vi "Push_Data_via_Public_Client.vi"(5 "Archive File?":bool[](array[boolean]), 6 "application reference":refnum<vi>, 7 "error in (no error)":errorcluster, 8 "Running on Server?":bool, 10 "Path of Files relative to EnFlo Data Root":path[](array[path])) -> (0 "error out":errorcluster, 3 "Error String":string)   [LabVIEW 2016]
uses:
  Anemometry/Anemometry Sub Vis/Globals/Constants_global.vi
  Sub VIs/Harvest_Global.vi
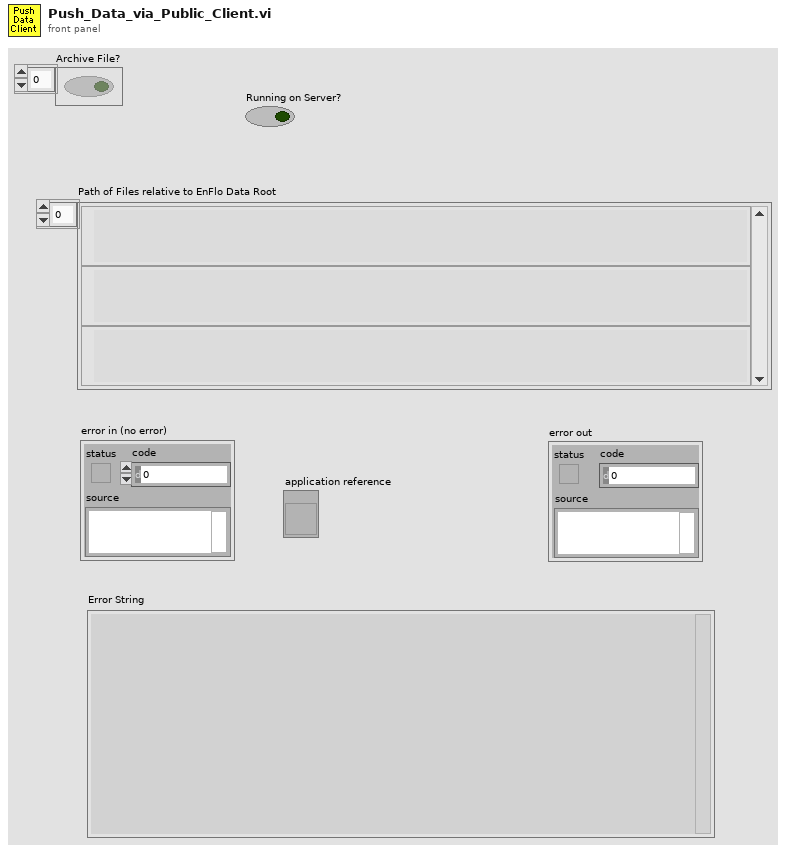
[diagram p1: front panel]
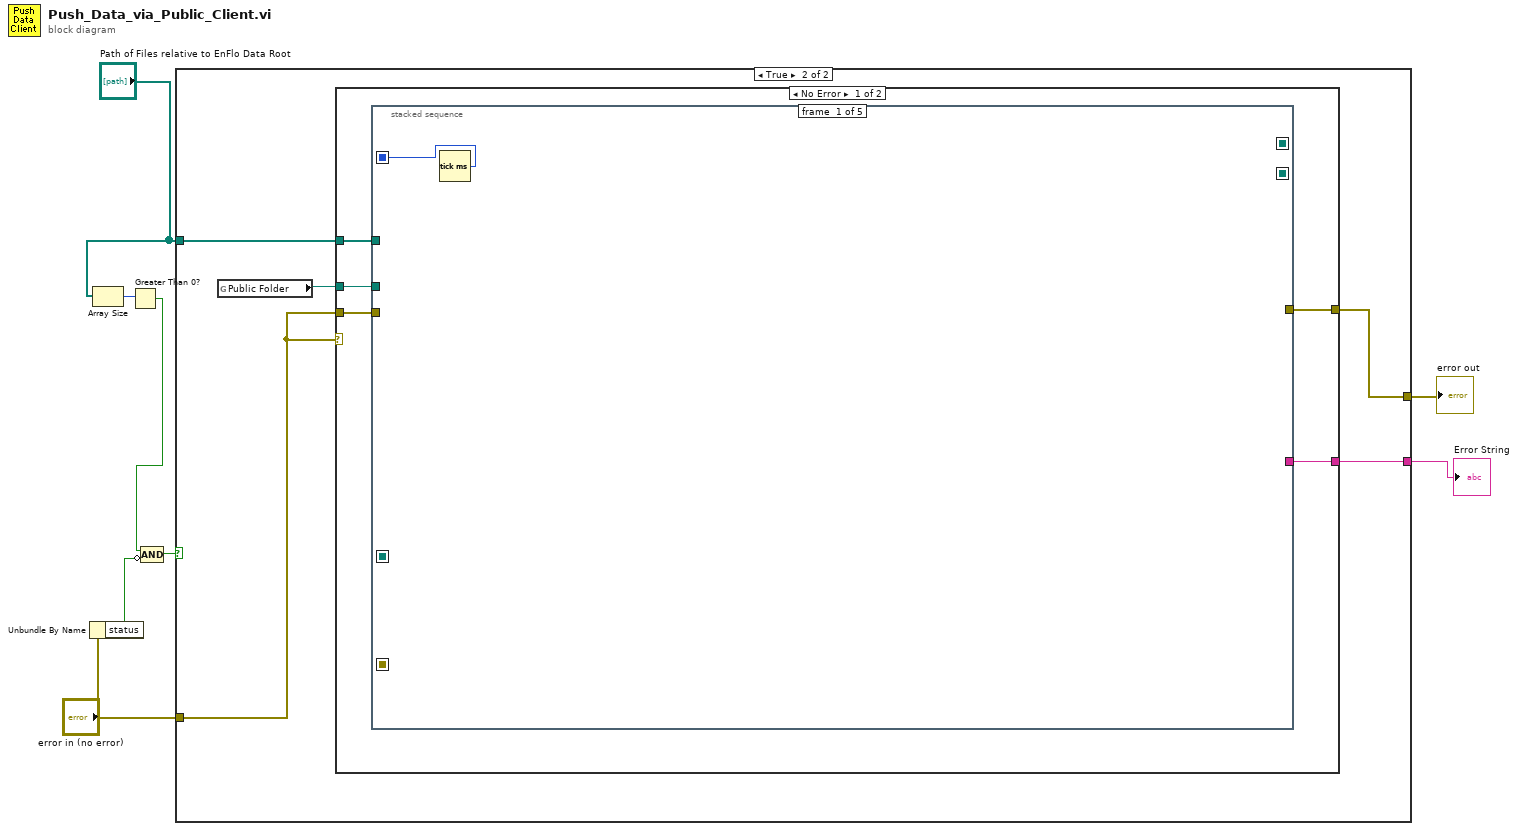
[diagram p0: block diagram]
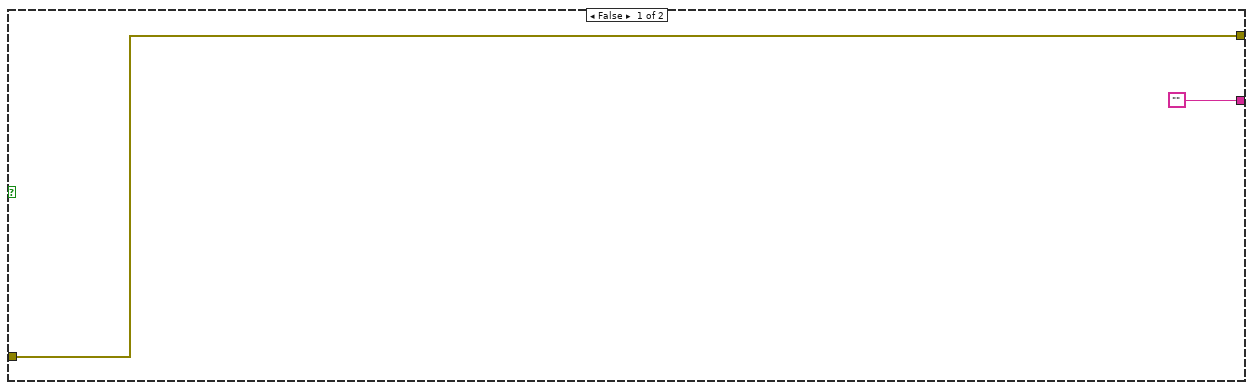
[diagram p2: hidden frame]
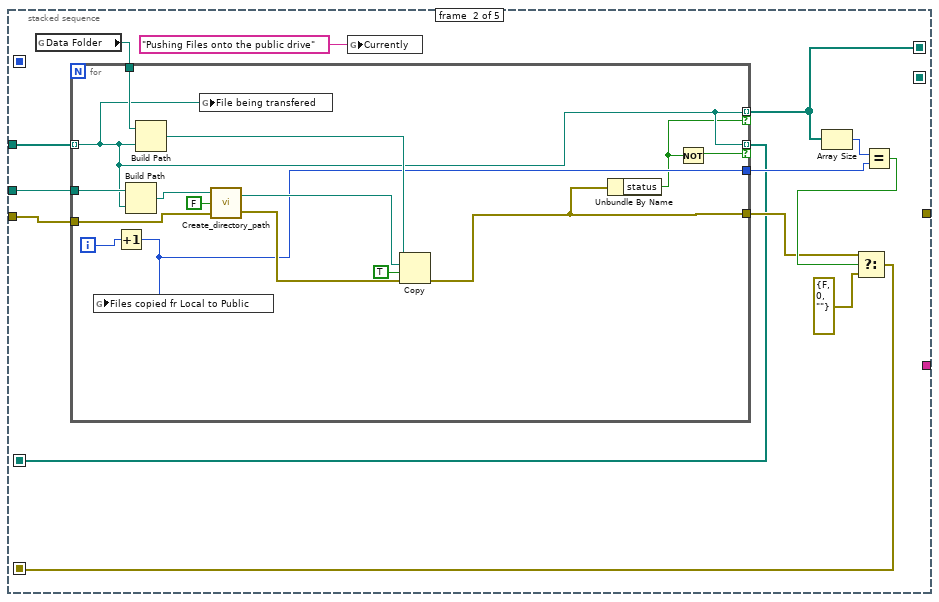
[diagram p3: hidden frame]
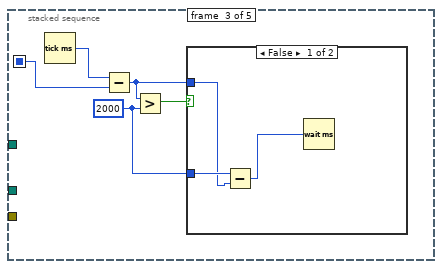
[diagram p4: hidden frame]
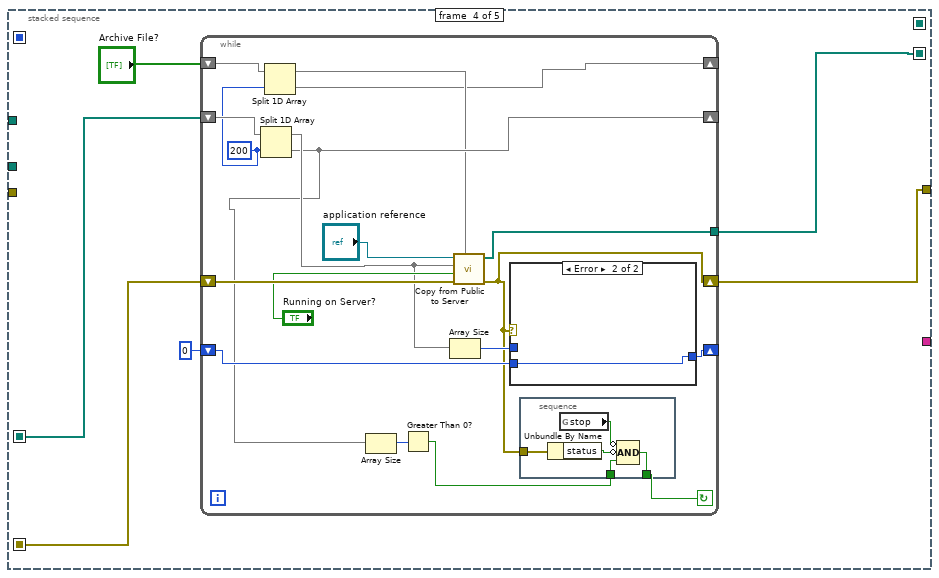
[diagram p6: hidden frame]
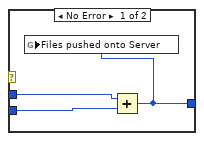
[diagram p7: hidden frame]
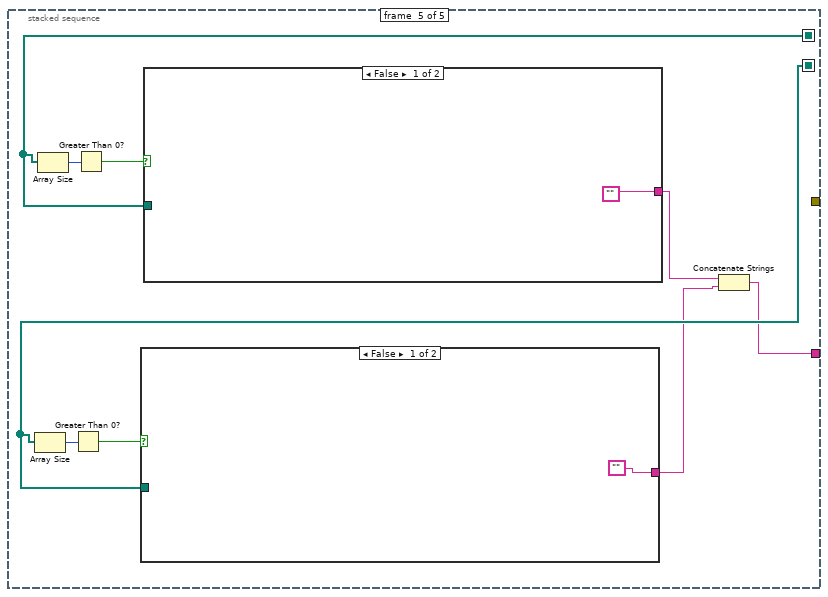
[diagram p8: hidden frame]
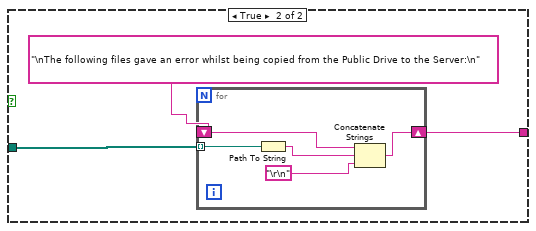
[diagram p9: hidden frame]
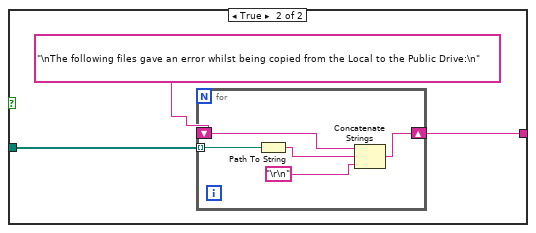
[diagram p10: hidden frame]
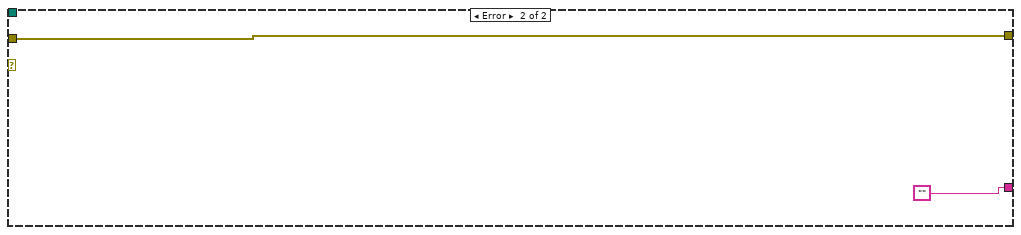
[diagram p11: hidden frame]
diagram:
  n1 = Unbundle By Name("error in (no error)") -> ("status"=w3:bool)
  n2 = Array Size(array="Path of Files relative to EnFlo Data Root") -> (size(s)=w6:i32)
  n3 = Greater Than 0?(x=w6) -> (x > 0?=w4:bool)
  n4 = Compound Arithmetic op=AND(w4, invert w3) -> (w2:bool)
  n5 = case shown="True" w2 {
    tunnel: [w10 w12] -> w8
    tunnel: "error in (no error)" -> [w10 w15]
    tunnel: "Path of Files relative to EnFlo Data Root" -> [_ w13]
    tunnel: ["" w11] -> w1
    frame False {
    }
    frame True {
      n6 = global read "Constants_global.vi" "Public Folder"() -> (w14:path)
      n7 = case shown="No Error" w15 {
        tunnel: [w17 w119] -> w12
        tunnel: w15 -> [w18 w119]
        tunnel: w13 -> [w20 _]
        tunnel: w14 -> [w19 _]
        tunnel: [w16 ""] -> w11
        frame No Error {
          n8 = stacked-sequence {
            seq-local: [w21 _ _ _ _] -> [_ _ w53 _ _]
            seq-local: [_ w24 _ _ _] -> [_ _ _ w63 _]
            seq-local: [_ w23 _ _ _] -> [_ _ _ _ w99]
            seq-local: [_ w22 _ _ _] -> [_ _ _ w59 _]
            seq-local: [_ _ _ w58 _] -> [_ _ _ _ w94]
            tunnel: w20 -> [_ w33 _ _ _]
            tunnel: w19 -> [_ w32 _ _ _]
            tunnel: w18 -> [_ w31 _ _ _]
            tunnel: [_ _ _ w62 _] -> w17
            tunnel: [_ _ _ _ w91] -> w16
            frame #0 {
              n9 = Tick Count (ms)() -> (millisecond timer value=w21:u32)
            }
            frame #1 {
              n10 = global read "Constants_global.vi" "Data Folder"() -> (w34:path)
              n11 = for {
                tunnel: w34 -> [w43]
                tunnel: w33 -> [w37] mode=indexing
                tunnel: w32 -> [w47]
                tunnel: w31 -> [w44]
                tunnel: [w40] -> w25
                tunnel: [w37] -> w23 mode=indexing if=w36
                tunnel: [w39] -> w28
                tunnel: [w37] -> w22 mode=indexing if=w35
                i -> [w42]
                n12 = Increment(x=w42) -> (x+1=w39:i32)
                n13 = global write "Harvest_Global.vi" "Files copied fr Local to Public"(w39) -> ()
                n14 = Build Path(base path=w47, name or relative path=w37) -> (appended path=w48:path)
                n15 = Build Path(base path=w43, name or relative path=w37) -> (appended path=w49:path)
                n16 = global write "Harvest_Global.vi" "File being transfered"(w37) -> ()
                n17 = call "Create_directory_path.vi"("error in (no error)"=w44, "Dialog Box"=FALSE, "Path name"=w48) -> ("error out"=w45:errorcluster, "Path name Out"=w46:path)
                n18 = Copy(8:w45, 9:TRUE ("overwrite (F)"), 10:w46, 11:w49) -> (0:w40:errorcluster)  [unwired: 1 in, 2 out]
                n19 = Unbundle By Name(w40) -> ("status"=w36:bool)
                n20 = Not(x=w36) -> (.not. x?=w35:bool)
              }
              n21 = global write "Harvest_Global.vi" "Currently"("Pushing Files onto the public drive" ("Currently Running")) -> ()
              n22 = Array Size(array=w23) -> (size(s)=w29:i32)
              n23 = Equal?(x=w29, y=w28) -> (x = y?=w26:bool)
              n24 = Select(t=w25, s=w26, f=errorcluster {"status"=FALSE, "code"=0, "source"=""} ("error out")) -> (s? t:f=w24:errorcluster)
            }
            frame #2 {
              w51 = u32 2000 ("y")
              n25 = Tick Count (ms)() -> (millisecond timer value=w54:u32)
              n26 = Subtract(x=w54, y=w53) -> (x-y=w50:u32)
              n27 = Greater?(x=w50, y=w51) -> (0:w52:bool)
              n28 = case shown="False" w52 {
                tunnel: w51 -> [w57 _]
                tunnel: w50 -> [w56 _]
                frame False {
                  n29 = Subtract(x=w57, y=w56) -> (x-y=w55:u32)
                  n30 = Wait (ms)(milliseconds to wait=w55) -> ()  [unwired: 1 out]
                }
                frame True {
                }
              }
            }
            frame #3 {
              n31 = while {
                shift-right: [w73] -> w62
                shift-left: w63 -> [w81]
                shift-right: [w72] -> _
                shift-left: w59 -> [w78]
                shift-right: [w75] -> _
                shift-left: 0 -> [w74]
                shift-right: [w65] -> _
                shift-left: "Archive File?" -> [w68]
                tunnel: [w64] -> w58
                stop <- w69 continue-if-true
                w67 = 200 ("index")
                n32 = Split 1D Array(array=w78, index=w67) -> (first subarray=w77:path[], second subarray=w72:path[])
                n33 = Split 1D Array(array=w68, index=w67) -> (first subarray=w66:bool[], second subarray=w65:bool[])
                n34 = Array Size(array=w72) -> (size(s)=w71:i32)
                n35 = Greater Than 0?(x=w71) -> (x > 0?=w70:bool)
                n36 = Array Size(array=w77) -> (size(s)=w76:i32)
                n37 = call "Copy from Public to Server.vi"("Archive File?"=w66, "error in (no error)"=w81, "Running on Server?"="Running on Server?", "Path of Files relative to EnFlo Data Root"=w77, "Application in"="application reference") -> ("error out"=w73:errorcluster, "Problem Files"=w64:path[])  [unwired: 5 in]
                n38 = case shown="Error" w73 {
                  tunnel: w76 -> [w89 _]
                  tunnel: [w87 w90] -> w75
                  tunnel: w74 -> [w88 w90]
                  frame No Error {
                    n39 = Add(x=w89, y=w88) -> (x+y=w87:i32)
                    n40 = global write "Harvest_Global.vi" "Files pushed onto Server"(w87) -> ()
                  }
                  frame Error {
                  }
                }
                n41 = stacked-sequence {
                  tunnel: [w85] -> w69
                  tunnel: w73 -> [w83]
                  tunnel: w70 -> [w82]
                  frame #0 {
                    n42 = Unbundle By Name(w83) -> ("status"=w86:bool)
                    n43 = global read "Harvest_Global.vi" "stop"() -> (w84:bool)
                    n44 = Compound Arithmetic op=AND(invert w84, invert w86, w82) -> (w85:bool)
                  }
                }
              }
            }
            frame #4 {
              n45 = Array Size(array=w94) -> (size(s)=w95:i32)
              n46 = Array Size(array=w99) -> (size(s)=w98:i32)
              n47 = Greater Than 0?(x=w95) -> (x > 0?=w96:bool)
              n48 = Greater Than 0?(x=w98) -> (x > 0?=w97:bool)
              n49 = case shown="False" w96 {
                tunnel: w94 -> [_ w103]
                tunnel: ["" w101] -> w92
                frame False {
                }
                frame True {
                  n50 = for {
                    tunnel: w103 -> [w108] mode=indexing
                    shift-right: [w105] -> w101
                    shift-left: "\nThe following files gave an error whilst being copied from the Public Drive to the Server:\n" -> [w104]
                    n51 = Path To String(path=w108) -> (string=w107:string)
                    n52 = Concatenate Strings(w104, w107, "\r\n") -> (w105:string)
                  }
                }
              }
              n53 = case shown="False" w97 {
                tunnel: w99 -> [_ w112]
                tunnel: ["" w110] -> w93
                frame False {
                }
                frame True {
                  n54 = for {
                    tunnel: w112 -> [w117] mode=indexing
                    shift-right: [w114] -> w110
                    shift-left: "\nThe following files gave an error whilst being copied from the Local to the Public Drive:\n" -> [w113]
                    n55 = Path To String(path=w117) -> (string=w116:string)
                    n56 = Concatenate Strings(w113, w116, "\r\n") -> (w114:string)
                  }
                }
              }
              n57 = Concatenate Strings(w93, w92) -> (w91:string)
            }
          }
        }
        frame Error {
        }
      }
    }
  }
  "error out" <- w8
  "Error String" <- w1
